vi "4.3.vi"() -> ()   [LabVIEW 2017]
panel:
  out "输出":dbl
  in  "输入":dbl
  in  "枚举":enum16{"平方", "平方根"}(ring)
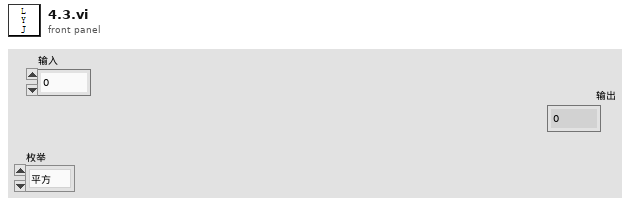
[diagram p1: front panel]
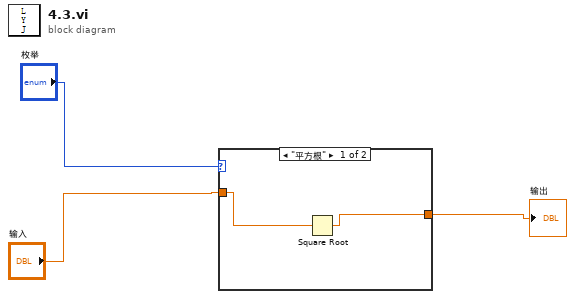
[diagram p0: block diagram]
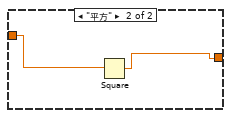
[diagram p2: hidden frame]
diagram:
  n1 = case shown="\"平方根\"" "枚举" {
    tunnel: "输入" -> [w5 w7]
    tunnel: [w4 w6] -> w1
    frame "平方根" {
      n2 = Square Root(x=w5) -> (sqrt(x)=w4:dbl)
    }
    frame "平方" {
      n3 = Square(x=w7) -> (x^2=w6:dbl)
    }
  }
  "输出" <- w1
